vi "AutonomousHatchPanelAndRocket.vi"   [LabVIEW 2018]
uses:
  Subsystems/Drive/driveShifterEnum.ctl
  Subsystems/HatchPanel/HatchPanelMotionEnum.ctl
types:
  T1 = typedef "HatchPanelMotionEnum.ctl" = enum16{"Retract", "Extend"}
  T2 = typedef "driveShifterEnum.ctl" = enum16{"Open", "Close"}
  T3 = enum16{"Right Cargo Ship", "Left Cargo Ship", "Left Rocket", "Right Rocket", "Scoring", "Right Acquire ", "Left Acquire"}
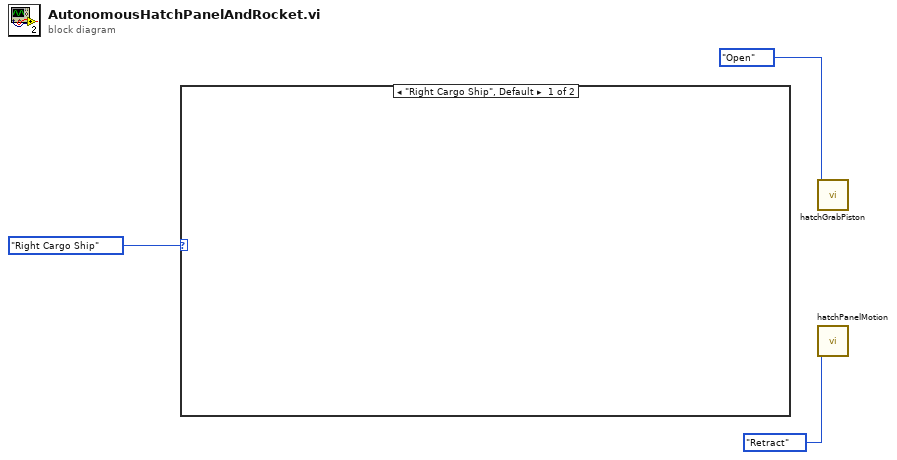
[diagram p0: block diagram]
diagram:
  n1 = case shown="\"Right Cargo Ship\", Default" T3."Right Cargo Ship" {
    frame "Right Cargo Ship", Default {
    }
    frame "Left Cargo Ship" {
    }
  }
  n2 = call "hatchGrabPiston.vi"(10:driveShifterEnum."Open") -> ()  [unwired: 11 in]
  n3 = call "hatchPanelMotion.vi"(10:HatchPanelMotionEnum."Retract") -> ()  [unwired: 11 in]
